vi "Set Channel Class.vi"(8 "error in":errorcluster, 11 "analog input Vrms mode in":refnum<class "Analog Input Vrms Mode.lvclass">) -> (0 "error out":errorcluster, 3 "analog input Vrms mode out":refnum<class "Analog Input Vrms Mode.lvclass">)   [LabVIEW 2019, in "Scan Engine Scripting.lvlib" / "Analog Input Vrms Mode.lvclass"]
uses:
  Analog Input Vrms Mode.lvclass
  Channel Classes/AI Vrms Channel/AI Vrms Channel.lvclass
  C:/Users/nitest/Desktop/Git 2019/niveristand-scan-engine-ethercat-custom-device/Custom Device Source/Scripting/Modules/Channel Classes/AI Channel/AI Channel.lvclass
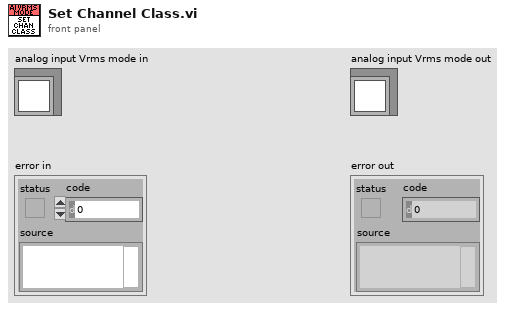
[diagram p1: front panel]
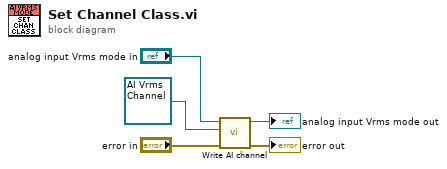
[diagram p0: block diagram]
diagram:
  n1 = call-dynamic "Write AI channel.vi"("error in"="error in", "analog input mode channel"=refnum<class "AI Vrms Channel.lvclass"> refnum ("Scan Engine Scripting.lvlib:AI Vrms Channel.lvclass"), "analog input mode in"="analog input Vrms mode in") -> ("error out"=→"error out":errorcluster, "analog input mode out"=→"analog input Vrms mode out":refnum<class "Analog Input Vrms Mode.lvclass">)  [unwired: 7 in]
